vi "Make Menu Tag.vi"(9 "String":string, 10 "Int":i32, 11 "Menu Tag":T1=enum."Create Channel Writer") -> (2 "Tag String":string, 3 "Label":string)   [LabVIEW 2022 SP3, in "FlexBlocks Support.lvlib"]
uses:
  FlexBlocks Support.lvlib
  Menu Tag.ctl
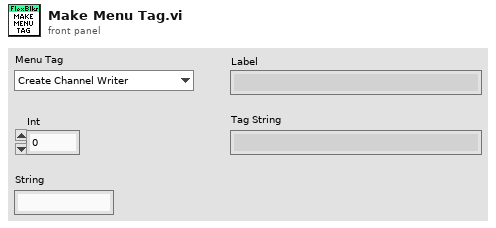
[diagram p1: front panel]
types:
  T1 = typedef "FlexBlocks Support.lvlib/Menu Tag.ctl" = enum16{"Unknown", "Create Channel Writer", "Create Lossy Reader", "Create Lossless Reader", "Create Event Reader", "Smol Mode"}
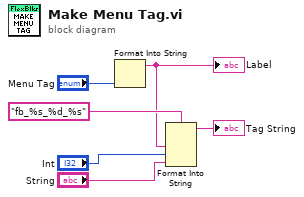
[diagram p0: block diagram]
diagram:
  n1 = Format Into String("Menu Tag") -> (resulting string=w1:string)  [unwired: 3 in, 1 out]
  "Label" <- w1
  n2 = Format Into String(format string="fb_%s_%d_%s", w1, "Int", "String") -> (resulting string=→"Tag String":string)  [unwired: 2 in, 1 out]
